vi "Close Toolbar.vi"(8 "error in (no error)":errorcluster, 11 "Toolbar Control in":refnum<class "Toolbar Control.lvclass">) -> (0 "error out":errorcluster)   [LabVIEW 2011, in "Toolbar Control.lvclass"]
doc: "This VI will close the toolbar, destroying any user events that have been created.\n\n-------------\nDeveloped by Brian Hoover (hooovahh)"
uses:
  Toolbar Control.lvclass
  Toolbar Control.lvclass/Toolbar Control.ctl
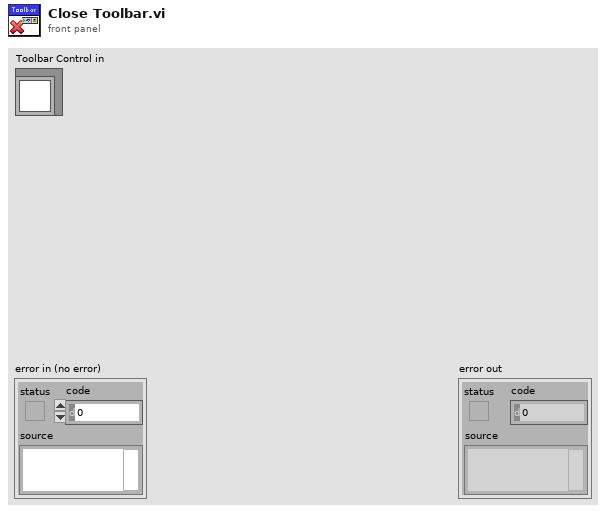
[diagram p1: front panel]
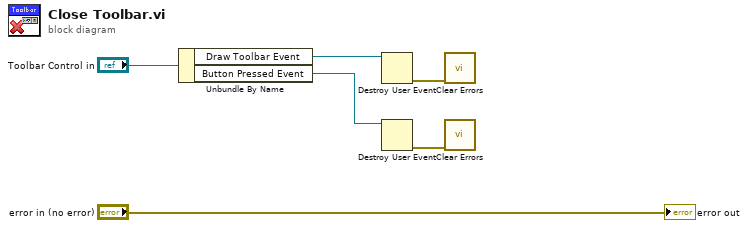
[diagram p0: block diagram]
diagram:
  n1 = Unbundle By Name("Toolbar Control in") -> ("Draw Toolbar Event"=w4:refnum<user-event>, "Button Pressed Event"=w3:refnum<user-event>)
  n2 = Destroy User Event(user event=w4) -> (error out=w1:errorcluster)  [unwired: 1 in]
  n3 = Destroy User Event(user event=w3) -> (error out=w2:errorcluster)  [unwired: 1 in]
  n4 = call <vilib>:"Clear Errors.vi"("error in (no error)"=w1) -> ()  [unwired: 6 in, 1 out]
  n5 = call <vilib>:"Clear Errors.vi"("error in (no error)"=w2) -> ()  [unwired: 6 in, 1 out]
  "error out" <- "error in (no error)"
